vi "set name.vi"(8 "error in (no error)":errorcluster caption="에러 입력(에러 없음)", 11 "PWL 입력":refnum<class "PWL.lvclass">) -> (0 "error out":errorcluster caption="에러 출력", 3 "PWL 출력":refnum<class "PWL.lvclass">)   [LabVIEW 2020, in "PWL.lvclass"]
uses:
  PWL.lvclass
  Waveform Gen/Waveform Gen.lvclass/Waveform Gen.ctl
  Waveform Obj/Waveform Obj.lvclass/Waveform Obj.ctl
  Waveform Gen/Accessors/Read frequency.vi
  Waveform Gen/Accessors/Read cycle.vi
  Waveform Gen/Accessors/Read scale.vi
  Waveform Obj/Accessors/Write name.vi
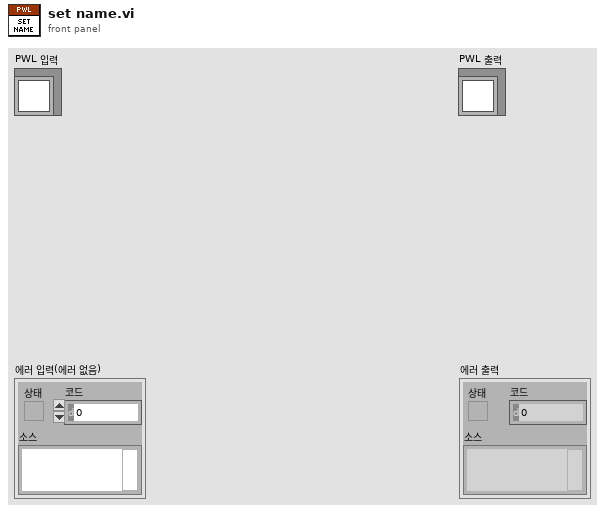
[diagram p1: front panel]
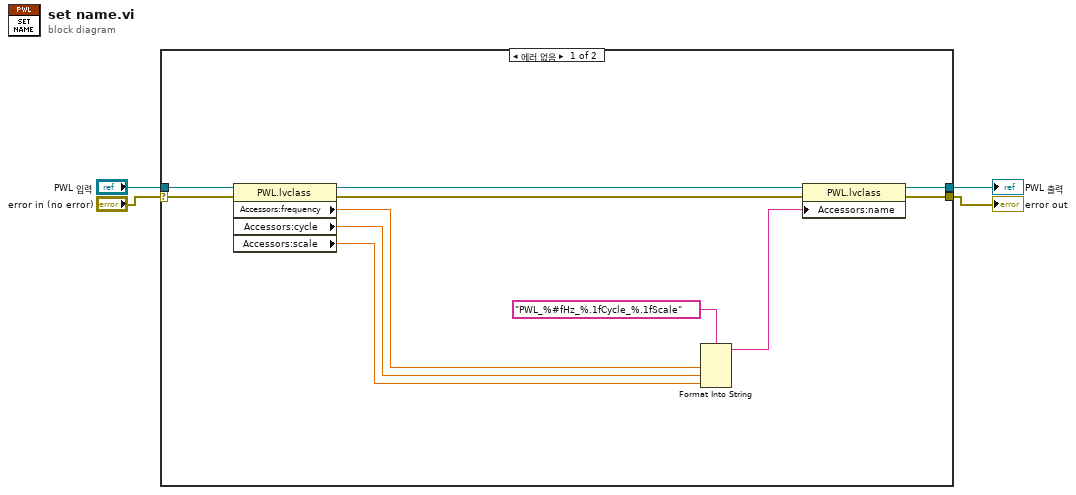
[diagram p0: block diagram]
diagram:
  n1 = case shown="에러 없음" "error in (no error)" {
    selector: "error in (no error)" -> [w11 w16]
    tunnel: "PWL 입력" -> [w10 w17]
    tunnel: [w9 w16] -> w4
    tunnel: [w8 w17] -> w3
    frame No Error {
      n2 = property class="PWL.lvclass"(reference=w10, error in=w11) -> (reference out=w7:refnum<class "PWL.lvclass">, error out=w5:errorcluster, "Accessors:frequency"=w14:dbl, "Accessors:cycle"=w13:dbl, "Accessors:scale"=w12:dbl)
      n3 = Format Into String(format string="PWL_%#fHz_%.1fCycle_%.1fScale" ("포맷 문자열"), w14, w13, w12) -> (resulting string=w6:string)  [unwired: 2 in, 1 out]
      n4 = property class="PWL.lvclass"(reference=w7, error in=w5, "Accessors:name"=w6) -> (reference out=w8:refnum<class "PWL.lvclass">, error out=w9:errorcluster)
    }
    frame Error {
    }
  }
  "error out" <- w4
  "PWL 출력" <- w3
